vi "AlliGator Subtract Background Image(s) v4.vi"(8 "error in (no error)":errorcluster, 9 "Background Gate Images, Min, Max & Sum 2":T1, 10 "Background Gate Images, Min, Max & Sum 1":T1, 11 "AlliGator IV DVR in":refnum<data-value>) -> (0 "error out":errorcluster, 3 "AlliGator IV DVR out":refnum<data-value>)   [LabVIEW 2021, in "AlliGator Files.lvlib"]
doc: "Computes background-subtracted single- or dual-channel dataset image structures."
uses:
  AlliGator Files.lvlib
  Internal Variables/AlliGator Internal Variables v2.ctl
  <vilib>/vision/Image Controls.llb/IMAQ Image.ctl
  Internal Variables/AlliGator Gate Image Set.ctl
  AlliGator FLI Dataset Type.ctl
  AlliGator Data Series Type.ctl
  Dual-Channel Datasets/AlliGator Dataset Channel.ctl
  Settings/AlliGator Gate Arithmetic.ctl
  Source Image/AlliGator Displayed Image.ctl
  Image/Named ROI Description.ctl
  Phasor Graph/AlliGator Decay Metadata v3.ctl
  Decay Analysis/Decay Preprocessing/AlliGator Decay Background Subtraction Info.ctl
  Decay Analysis/Decay Preprocessing/AlliGator Baseline Subtraction Method.ctl
  Graphs/XY Graph/XY Graph Plot Shift Parameters.ctl
  Graphs/XY Graph/XY Graph Plot Shift Method.ctl
  Decay Analysis/Decay Preprocessing/AlliGator Decay Extrapolation Parameters.ctl
  Phasor/Calibration Phasor (m, phi).ctl
  Phasor/Phasor Reference Series.ctl
  Phasor/Phasor Calibration Map v2.ctl
  Phasor/Phasor (g, s).ctl
  Phasor Graph/AlliGator Raw Phasor Plot Data v5.ctl
  Phasor/Phasor Standard Deviation Options.ctl
  Phasor Plot/AlliGator Phasor Multi-Harmonic Data.ctl
  Phasor/Phasor Harmonic Data.ctl
  Decay Fit Parameter Map/AlliGator Decay Fit Options & Parameters v4.ctl
  Fits/IRF(X)PSED/Decay Fit Options v4.ctl
  Fits/Decay Convolution/Decay Model.ctl
  Fits/Residual Type.ctl
  Fits/IRF(X)PSED/Fit Weights Type v2.ctl
  Fits/Non-linear Fitting Method v2.ctl
  Fits/Fit Calculation Method.ctl
  Fits/Non-linear Fitting Algorithm.ctl
  Decay Analysis/Decay Fit/AlliGator Decay Fit Parameter Constraints 2.ctl
  Fits/IRF(X)PSED/Decay Fit Parameters In List.ctl
  Fits/IRF(X)PSED/MLE Baseline Offset Type.ctl
  Decay Analysis/Decay Preprocessing/AlliGator Decay Preprocessing Parameters.ctl
  Fits/IRF(X)PSED/Decay Fit Parameters & Derived Quantities List v2.ctl
  Fits/IRF(X)PSED/Decay Fit Result Constraint.ctl
  Decay Fit Parameter Map/AlliGator Parameter Maps Data.ctl
  Globals, Variables, Constants/AlliGator Variables List.ctl
  Variant/Variant to Data/Variant to U16.vi
  <vilib>/Utility/error.llb/Error Cluster From Error Code.vi
  <vilib>/ErrorRing/Error Ring.xnode
  <vilib>/vision/NI_Vision_Development_Module.lvlib
  Image/Image.lvlib
  Error/Error.lvlib
  Strings/Strings.lvlib
  Globals, Variables, Constants/AlliGator Globals, Variables & Constants.lvlib
  Dual-Channel Datasets/AlliGator Dual-Channel Datasets.lvlib
  Variant/Variant to Data/Variant to Data.lvlib
  Phasor/Phasor.lvlib
  Internal Variables/AlliGator Internal Variables.lvlib
  Phasor Graph/AlliGator Phasor Graph.lvlib
  Decay Analysis/Decay Preprocessing/AlliGator Decay Preprocessing.lvlib
  Graphs/XY Graph/XY Graph Add-Ons.lvlib
  Phasor Plot/AlliGator Phasor Plot.lvlib
  Source Image/AlliGator Source Image.lvlib
  Fits/Fits.lvlib
  Decay Analysis/Decay Fit/AlliGator Decay Fit.lvlib
  Settings/AlliGator Settings.lvlib
  Decay Fit Parameter Map/AlliGator Decay Fit Parameter Map.lvlib
panel:
  # "see the AlliGator License on the block diagram (Ctrl+E or Window:Show Block Diagram)"
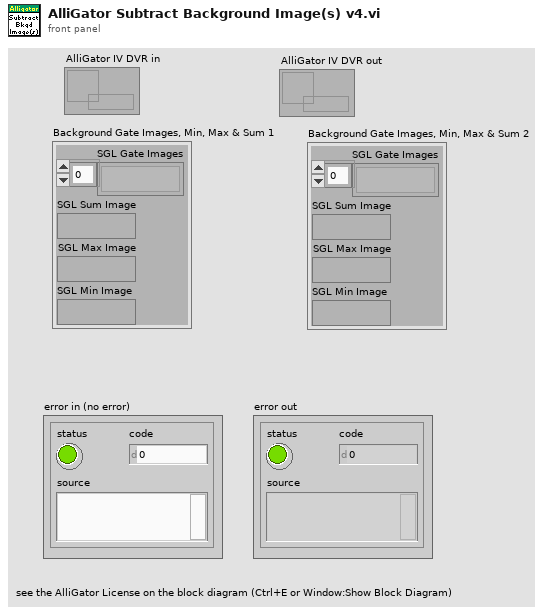
[diagram p1: front panel]
types:
  T1 = typedef "AlliGator Internal Variables.lvlib/AlliGator Gate Image Set.ctl" = cluster{"SGL Gate Images":T2[], "SGL Sum Image":T2, "SGL Max Image":T2, "SGL Min Image":T2}
  T2 = typedef "IMAQ Image.ctl" = refnum<image>
  T3 = typedef "Image Type" = u32
  T4 = typedef "AlliGator Globals, Variables & Constants.lvlib/AlliGator Variables List.ctl" = enum16{"---- GUI ----", "GUI:Initialization Status", "GUI:State Indicators Refnum", "GUI:Original AlliGator Menu Items", "GUI:Current Action Loop State", "GUI:Script in progress", "GUI:Playback", "GUI:Loop Playback", "GUI:Search ROI Used", "GUI:Search ROI", "Decay Graph Max Legend Size", "Intensity Graph Max Legend Size", "Decay Statistics Graph Max Legend Size", "Phasor Graph Max Legend Size", "Phasor Ratio Graph Max Legend Size", "Lifetime Graph Max Legend Size", "---- Files ----", "Files:Export Dataset Frames as Individual Files", "Files:Show Batch Export Help Balloons", "Files:Frames in Dataset", "Files:ptu File Frame Start Indices", "Files:Current Frame in Dataset", "Files:Current Frame Timestamp", "Files:Dataset Loaded", "Files:Dataset Metadata", "Files:Dataset Channel", "Files:Dataset Data Description", "Files:Background Dataset Metadata", "Files:Background Dataset Channel", "Files:Background Dataset Data Description", "Files:Background File Subtraction", "Files:Background File Path", "Files:Background File Pile-up Correction", "Files:Background File Pixel Well Capacity", "Files:Background File Scaling Factor", "Files:Current Dataset Load Settings", "Files:Dataset Path", "Files:ICCD-specific Information", "Files:Macrotime Gate Separation", "------ Python Plugins ------", "Python Plugins:Information", "Python Plugins:Python Session", "Python Plugins:Valid Python Session?", "---- Source Image ----", "Source Image:ROIs", "Source Image:Current ROI", "Source Image:ROI Event Refnum", "X_Source Image:Display Range", "X_Source Image:Palette Information", "X_Source Image:Type of Displayed Image", "X_Time Gate Slider", "Source Image:Palette List", "Source Image:Scale", "Source Image:ROI Overlay Color", "Source Image:Overlay to Erase", "Source Image:Is Displayed Image Accumulated", "Source Image:White Light Image Modified", "Source Image:Mask Image Modified", "---- Image Profile Window ----", "Image Profile:Window Event Refnum", "Image Profile:IntensityType", "Image Profile:Intensity Average Type", "Image Profile:Intensity-weighted SDV", "Image Profile:Box Profile Type", "Image Profile:Window Open", "Image Profile:Plotted Fit Parameter", "------ Phasor Graph -------", "Phasor Graph:Show Line", "---- Phasor Plot ---", "Phasor Plot:Parameters Changed", "Phasor Plot:FLI Dataset Modified since last Calculation", "Phasor Harmonics Data", "Selected Phasor Harmonics", "Phasor Harmonic Manager Event Refnum", "Phasor Plot:ROIs", "Phasor Plot:Current ROI", "Phasor Plot:ROI Event Refnum", "Phasor Plot:Image Reference Points", "Phasor Plot:Computed", "Phasor Plot:Palette Information", "Phasor Plot:Palette List", "Phasor Plot:Phasor Ratio Palette Information", "Phasor Plot:Phasor Ratio Palette List", "Phasor Plot:Image Scale", "Phasor Plot:Image Overlay to Erase", "Phasor Plot:Image Elements to Update", "Phasor Plot:Current Calculation Parameters", "Phasor Plot:Current Calibration Options", "Phasor Plot:Reset Cumulated Phasor Plot", "Phasor Plot:Reference 1", "Phasor Plot:Lifetime Reference 1", "Phasor Plot:Reference 1 Frequency", "Phasor Plot:Reference 2", "Phasor Plot:Lifetime Reference 2", "Phasor Plot:Reference 2 Frequency", "---- Decay Analysis ----", "Number of Selected Decays to Fit", "LS Fit Results", "LAR Fit Results", "BS Fit Results", "Last Decay Max - Min", "Best Fit Parameters", "Best Fit Parameter Names", "Actual Size X", "Actual Size Y", "Binning X", "Binning Y", "Actual # Gates", "Dataset Number", "Gates to...", "Gates Skipped", "Gates to keep", "Gate Step", "Gate Separation", "Reversed Gates", "Pile-up Correction", "Pixel Well Capacity", "Background Subtracted", "Background Subtraction Method", "Background Definition Range", "Background File (deprecated)", "Number of Dataset Accumulated", "Array of Accumulated Dataset Paths", "Do Averaged Datasets", "Destination File Path", "Process Plot Target", "Use 1/D as Phasor Frequency", "---- Decay Fit Parameter Map -----", "Decay Fit Parameter Map:Palette Information", "Decay Fit Parameter Map:Palette List", "Decay Fit Parameter Map:X Resolution", "Decay Fit Parameter Map:Y Resolution", "Decay Fit Parameter Map:Use Decay Fit Result Constraints", "Decay Fit Parameter Map:Decay Fit Result Constraints", "Decay Fit Parameter Map:Decay Fit Result Constraints Applied", "---- Parameter Map ----", "Parameter Map:Palette Information", "Parameter Map:Palette List", "------- Local Decay Window ---------", "Local Decay Graph Window:Event Refnum", "Local Decay Graph Window:Use normalized IRF for convolution", "----- Miscellaneous ----", "Misc:Skippable Dialog Windows Status"}
  T5 = typedef "AlliGator Internal Variables.lvlib/AlliGator Internal Variables v2.ctl" = cluster{"----------------------------- Images -----------------------------":u8, "Displayed Image":T2, "White Light Image":T2, "Mask Image":T2, "ROI Mask Image":T2, "Current Dataset Images 1":T1, "Background Dataset Images 1":T1, "Current Dataset Images 2":T1, "Background Dataset Images 2":T1, "Current Dataset Arithmetic Images":T1, "Accumulated Dataset Images 1":T1, "Accumulated Dataset Images 2":T1, "Accumulated Dataset Arithmetic Images":T1, "----------------------------- File Paths -----------------------------":u8, "Phasor Plot Image":T2, "Decay Fit Parameter Map Image":T2, "Parameter Map Image":T2, "Single Data Point Path":path, "White Light Image Path":path, "Mask Image Path":path, "Time-Series Folder":path, "[Time-Series Paths]":path[], "----------------------------- FLI Dataset -----------------------------":u8, "Current Dataset":i32, "Single Dataset Type":T6, "Current Folder":string, "AlliGator Data Series Type":T7, "# Datasets":i32, "Dual-Channel Dataset":bool, "Selected Channel Name":string, "Dataset Channel":T8, "Channel Arithmetic":T9, "Dual-Channel Background Dataset":bool, "Background Channel":T8, "Dual-Channel Accumulated Dataset":bool, "Start Time":dbl, "[Time-Series Timestamps]":dbl[], "[Intensity Corrections]":dbl[], "Time Series Script":bool, "Type of Displayed Image":T10, "Gate Image Slide":u16, "# Gates":i32, "ROIs":T11[], "----------------------------- Decays -----------------------------":u8, "ROI Decay":cluster{"t Array":dbl[], "I Array":dbl[]}, "Valid Decay":bool, "Decay  Metadata":T13, "Reference Decay Plot Name":string, "Reference Decay":cluster{"t Array":dbl[], "I Array":dbl[]}, "Decay Shift Plot":cluster{"Time Stamps":dbl[], "Decay Shifts":dbl[]}, "[Decays Max Values]":sgl[], "[Decays Min Values]":sgl[], "----------------------------- Calibration -----------------------------":u8, "Calibration Phasor":T19, "Calibration Phasor Series":T20, "Phasor Calibration Map":T21, "Calibration Map MD5 Digest":string, "----------------------------- Phasor Graph -----------------------------":u8, "Last Raw Phasor":T22, "Last Calibrated Phasor":T22, "Last Calibrated Phasor SDV":T22, "Phasor Graph:Phasor Plot":cluster{"g Array":dbl[], "s Array":dbl[]}, "Phasor Graph:Phasor SDV Plot":cluster{"g Array":dbl[], "s Array":dbl[]}, "[Phasor Graph:Raw Phasor Plots]":T23[], "Phasor Plot locked to Ref 1":i32, "[Phasor Plot(s) locked to Ref 1]":i32[], "[Phasor Plot(s) locked to Ref 2]":i32[], "[Pixel Phasors]":T22[], "----------------------------- Phasor Plot -----------------------------":u8, "[[Sum Image]]":dbl[][], "[[CSG Phasors]]":csg[][], "[[Valid Pixel?]]":bool[][], "[[Phasor Ratios]]":dbl[][], "[[Average Lifetimes]]":dbl[][], "Amplitude Weighted Average Lifetime":bool, "I/m/phi Dataset":cluster{"I/m/phi Dataset?":bool, "Base Frequency":dbl[unit], "Harmonic Orders":u8[]}, "Multi Phasor Plot Data":T25, "----------------------------- Decay Fit Parameter Map -----------------------------":u8, "Decay Fit Options & Parameters":T27, "Fit Options: Decay Preprocessing Parameters":T38, "Fit Options: Reference Decay":cluster{"t Array":dbl[], "I Array":dbl[]}, "Is Full Image Parameters Map":bool, "Is Single-Pixels Parameters Map":bool, "NLSF Parameters Map X Resolution":i32, "NLSF Parameters Map Y Resolution":i32, "[Single Decay Fit Parameters]":dbl[], "Fit Model":T29, "[[Multiple Decays Fit Parameters]]":dbl[][], "[[Multiple Decays Fit Parameter SDVs]]":dbl[][], "[[IRFs]]":dbl[][], "[ROI Descriptors]":T12[], "IRF Array Time Axis":dbl[], "Decay Array Time Axis":dbl[], "[Decay Fit Parameter Names]":T39[], "[Decay Sum]":dbl[], "Array of Decay Fit Result Constraints":T40[], "Selected ROIs Array":bool[], "----------------------------- Parameter Maps -----------------------------":u8, "[Map Set Names]":string[], "[Parameter Maps]":T41[], "[[User-defined Quantities]]":dbl[][], "User-defined Quantity":string}
  T6 = typedef "AlliGator Files.lvlib/AlliGator FLI Dataset Type.ctl" = enum16{"HDF5 FLI Dataset", "Gate Image Folder", ".sdt FLI Dataset (Becker & Hickl)", ".ptu FLI Dataset (PicoQuant)", "SS1 FLI Dataset", "SS2 FLI Dataset", "I/m/phi Dataset", ".bin FLI Dataset (PicoQuant Binned)", ".bin FLI Dataset (Piccolo Binned)", ".mat FLI Dataset"}
  T7 = typedef "AlliGator Files.lvlib/AlliGator Data Series Type.ctl" = enum16{"Not a Supported Series", "Gate Images Folder Series", "SwissSPAD 2 Dataset Series", "B&H FLI Dataset Series", "PicoQuant PTU FLI Dataset Series", "PicoQuant BIN FLI Dataset Series", "Piccolo hist BIN FLI Dataset Series", "HDF5 FLI Dataset Series"}
  T8 = typedef "AlliGator Dual-Channel Datasets.lvlib/AlliGator Dataset Channel.ctl" = enum16{"G2", "INT"}
  T9 = typedef "AlliGator Settings.lvlib/AlliGator Gate Arithmetic.ctl" = enum16{"None", "INT-G2", "G2/INT*<INT>", "(1 - G2/INT)*<INT>"}
  T10 = typedef "AlliGator Source Image.lvlib/AlliGator Displayed Image.ctl" = enum16{"Single Gate", "Sum of All Gates", "Max of All Gates", "Min of All Gates", "-", "White Ligth Image", "Mask Image"}
  T11 = typedef "Image.lvlib/Named ROI Description.ctl" = cluster{"ROI Descriptor":T12, "ROI Name":string, "Overlay Color":u32}
  T12 = typedef "ROI Descriptor" = cluster{"Global Rectangle":i32[], "Contours":cluster{"ID":enum32{"External", "Internal"}, "Type":u32, "Coordinates":i32[]}[]}
  T13 = typedef "AlliGator Phasor Graph.lvlib/AlliGator Decay Metadata v3.ctl" = cluster{"ROI Descriptor":T12, "ROI Center":cluster{"X":i32, "Y":i32}, "Decay Background Subtraction Info":T14, "Decay Reverted":bool, "Decay Smoothened":bool, "Decay Straightened":bool, "Fitted Tau (Decay Straightening)":dbl, "Decay Shift Parameters":T16, "Decay Shifted":bool, "Decay Extrapolated":bool, "Decay Extrapolation Parameters":T18, "Decay Normalized":bool, "Fold Decay":bool, "# Folds":u32}
  T14 = typedef "AlliGator Decay Preprocessing.lvlib/AlliGator Decay Background Subtraction Info.ctl" = cluster{"Laser Period":dbl[unit], "Gate Duration":dbl[unit], "Baseline Subtraction Method":T15, "Background Definition Range":cluster{"Min Gate":dbl[unit], "Max Gate":dbl[unit]}, "Total Intensity w/o Bkgd Subtraction":dbl, "Bkgd-subtracted Intensity (exp)":dbl, "# Data Points":i32, "Background/Gate":dbl, "Fitted Lifetime":dbl[unit], "Bkgd-subtracted Intensity (theo)":dbl}
  T15 = typedef "AlliGator Decay Preprocessing.lvlib/AlliGator Baseline Subtraction Method.ctl" = enum16{"Mean", "Min", "Square Gated Single-Exponential", "File", "Constant"}
  T16 = typedef "XY Graph Add-Ons.lvlib/XY Graph Plot Shift Parameters.ctl" = cluster{"Type":T17, "Shift":dbl[unit], "Threshold":dbl, "Rotate":bool}
  T17 = typedef "XY Graph Add-Ons.lvlib/XY Graph Plot Shift Method.ctl" = enum16{"Default", "CFD", "Threshold", "Cross-Correlation"}
  T18 = typedef "AlliGator Decay Preprocessing.lvlib/AlliGator Decay Extrapolation Parameters.ctl" = cluster{"Additional Points":u32, "Head Fraction":dbl, "Fitted Tau":dbl, "Use Periodicity":bool, "Use Cursors":bool, "Tail Fraction":dbl}
  T19 = typedef "Phasor.lvlib/Calibration Phasor (m, phi).ctl" = cluster{"m":dbl, "phi":dbl, "Phasor Frequency":dbl[unit], "Reference Lifetime":dbl[unit]}
  T20 = typedef "Phasor.lvlib/Phasor Reference Series.ctl" = cluster{"m Array":dbl[], "phi Array":dbl[], "Phasor Frequency":dbl[unit], "Calibration Lifetime":dbl[unit]}
  T21 = typedef "Phasor.lvlib/Phasor Calibration Map v2.ctl" = cluster{"Phasor Frequency":dbl[unit], "Calibration Lifetime":dbl[unit], "ROI Centers":cluster{"X":i32, "Y":i32}[], "ROI Descriptors":T12[], "Map Resolution X":i32, "Map Resolution Y":i32, "z Array":cdb[]}
  T22 = typedef "Phasor.lvlib/Phasor (g, s).ctl" = cluster{"g":dbl, "s":dbl}
  T23 = typedef "AlliGator Phasor Graph.lvlib/AlliGator Raw Phasor Plot Data v5.ctl" = cluster{"Phasor Plot Name":string, "Raw Phasor Plot":T22[], "Phasor Frequency":dbl[unit], "[Decay Metadata]":T13[], "Raw Phasor Plot SDV":T22[], "Phasor SDV Options":T24, "[Calibration Phasor]":T19[], "Intensity Array":dbl[]}
  T24 = typedef "Phasor.lvlib/Phasor Standard Deviation Options.ctl" = cluster{"Compute Estimated SDV":bool, "# Replicas":u32, "Use Estimated Average Phasor":bool}
  T25 = typedef "AlliGator Phasor Plot.lvlib/AlliGator Phasor Multi-Harmonic Data.ctl" = cluster{"Base Frequency":dbl[unit], "# Harmonics":u8, "Harmonic Orders":u8[], "Phasor Plot Settings Checksum":u64, "Phasor Harmonic Data Array":T26[]}
  T26 = typedef "Phasor.lvlib/Phasor Harmonic Data.ctl" = cluster{"Phasor Harmonic Name":string, "Phasor Plot Settings Checksum":u64, "Phasor Frequency":dbl[unit], "Base Frequency":dbl[unit], "Harmonic Order":u8, "Phasor Plot Parameters":string, "Phasor Array [[CSG]]":csg[][], "Dataset File Path":path}
  T27 = typedef "AlliGator Decay Fit Parameter Map.lvlib/AlliGator Decay Fit Options & Parameters v4.ctl" = cluster{"SYNC Period":dbl[unit], "Fit Options":T28, "Fit Parameter Constraints":T35[], "MLE Baseline Offset":dbl, "MLE Baseline Offset Type":T37}
  T28 = typedef "Fits.lvlib/Decay Fit Options v4.ctl" = cluster{"Show Fit Residuals":bool, "Fit Model":T29, "Residual Type":T30, "Max Decay Percentile":dbl, "Min Decay Percentile":dbl, "Show Full Decay":bool, "Weights":T31, "Fitting Method":T32, "Compute Parameter Uncertainties":bool, "Periodic Boundaries":bool, "Model Calculation":T33, "Period":dbl[unit], "Termination Criteria":cluster{"Max Iterations":i32, "Max Function Calls":i32, "Max Time":dbl[unit], "Function Tolerance":dbl, "Parameter Tolerance":dbl, "Gradient Tolerance":dbl, "Min Lambda":dbl, "Max Lambda":dbl, "Initial Tick Count":u32}, "Offset Resolution":dbl[unit], "Use Local IRF":bool, "Fitting Algorithm":T34, "Show Confidence Interval ":bool, "Confidence Level":dbl}
  T29 = typedef "Fits.lvlib/Decay Model.ctl" = enum16{"1-Exponential", "2-Exponentials"}
  T30 = typedef "Fits.lvlib/Residual Type.ctl" = enum16{"Standard", "Normalized", "Reduced"}
  T31 = typedef "Fits.lvlib/Fit Weights Type v2.ctl" = enum16{"Unweighted", "1/Variance (Neyman)", "1/Variance (Pearson)", "Best of All"}
  T32 = typedef "Fits.lvlib/Non-linear Fitting Method v2.ctl" = enum16{"Least Square", "Least Absolute Residual", "Bisquare", "MLE", "-", "Best of All"}
  T33 = typedef "Fits.lvlib/Fit Calculation Method.ctl" = enum16{"Simulation", "Convolution", "Integration"}
  T34 = typedef "Fits.lvlib/Non-linear Fitting Algorithm.ctl" = enum16{"Levenberg-Marquardt", "Trust-Region Dogleg"}
  T35 = typedef "AlliGator Decay Fit.lvlib/AlliGator Decay Fit Parameter Constraints 2.ctl" = cluster{"Fit Parameter":T36, "Min Value":dbl, "Max Value":dbl, "Global":bool, "Used":bool}
  T36 = typedef "Fits.lvlib/Decay Fit Parameters In List.ctl" = enum16{"Offset", "Baseline", "A_1", "tau_1", "A_2", "tau_2"}
  T37 = typedef "Fits.lvlib/MLE Baseline Offset Type.ctl" = enum32{"Absolute", "Percentage"}
  T38 = typedef "AlliGator Decay Preprocessing.lvlib/AlliGator Decay Preprocessing Parameters.ctl" = cluster{"Background Subtraction":bool, "Straighten Decay":bool, "Reverse Gates":bool, "1-Normalized Decay":bool, "Smoothen Decay":bool, "Smoothing Parameter":dbl, "Shift Decay":bool, "Decay Shift Parameters":T16, "Extrapolate Decay":bool, "Additional Points":u32, "Head Fraction":dbl, "Pixel-Normalize Decay":bool, "Use Periodicity":bool, "Use Cursors":bool, "Tail Fraction":dbl, "Use Decay Pre-Processing":bool, "Fold Decay":bool, "# Folds":u32, "[0-1]-Normalized Decay":bool}
  T39 = typedef "Fits.lvlib/Decay Fit Parameters & Derived Quantities List v2.ctl" = enum16{"Offset", "Baseline", "A_1", "tau_1", "A_2", "tau_2", "<tau>_a", "f1_a", "f2_a", "<tau>_i", "f1_i", "f2_i", "-", "R^2", "Chi^2"}
  T40 = typedef "Fits.lvlib/Decay Fit Result Constraint.ctl" = cluster{"Fit Parameter":enum16{"Offset", "Baseline", "A_1", "tau_1", "A_2", "tau_2", "<tau>_a", "f1_a", "f2_a", "<tau>_i", "f1_i", "f2_i", "-", "R^2", "Chi^2", "Max Relative Residual", "<Residual ACF>", "Residual ACF SDV", "tau_2/tau_1"}, "Min Value":dbl, "Max Value":dbl, "Use Constraint":bool}
  T41 = typedef "AlliGator Decay Fit Parameter Map.lvlib/AlliGator Parameter Maps Data.ctl" = cluster{"Map Set Name":string, "[Parameter Names]":string[], "[[Parameters]]":dbl[][], "[[Parameter SDVs]]":dbl[][], "Decay Array Time Axis":dbl[], "[[IRFs]]":dbl[][], "IRF Array Time Axis":dbl[], "X Resolution":i32, "Y Resolution":i32, "Intensity Array":dbl[]}
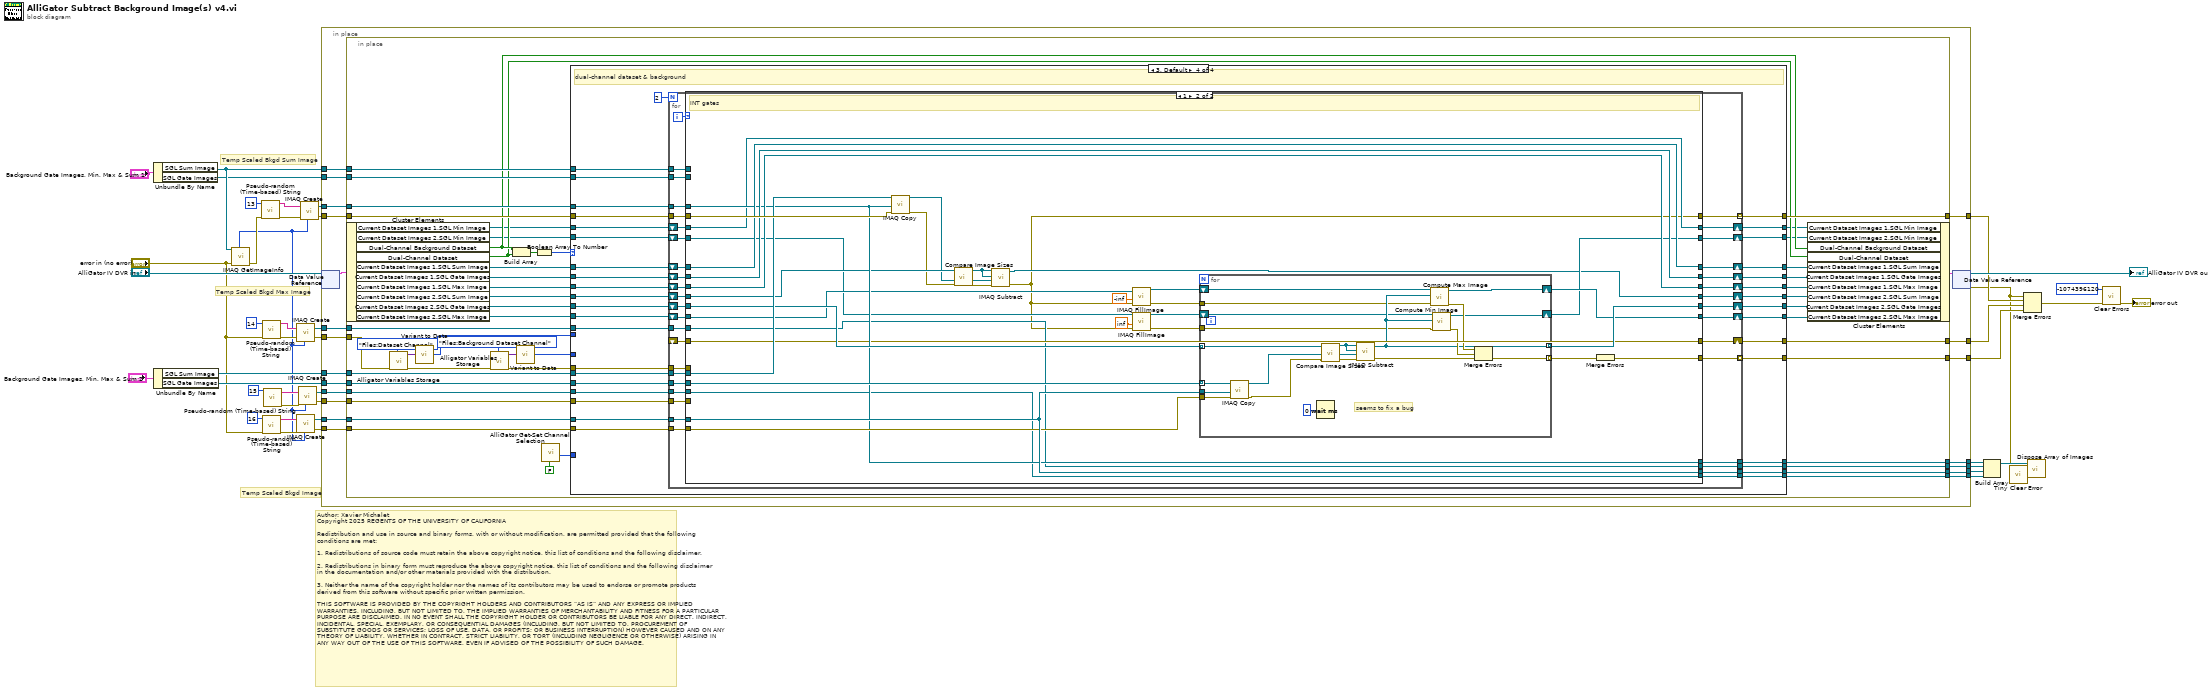
[diagram p0: block diagram]
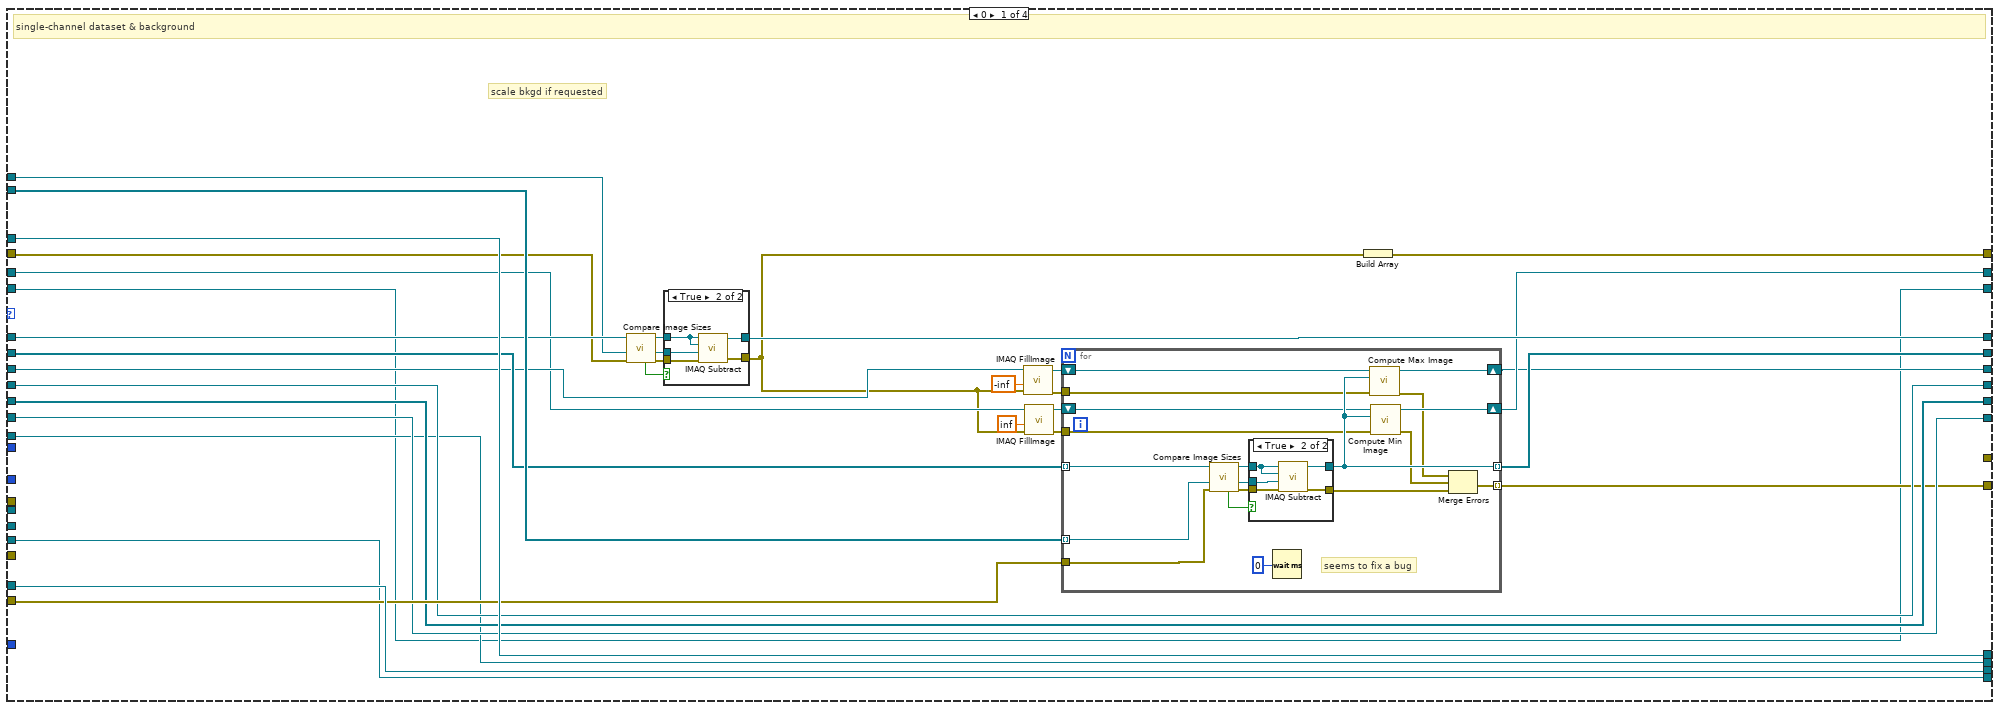
[diagram p2: hidden frame]
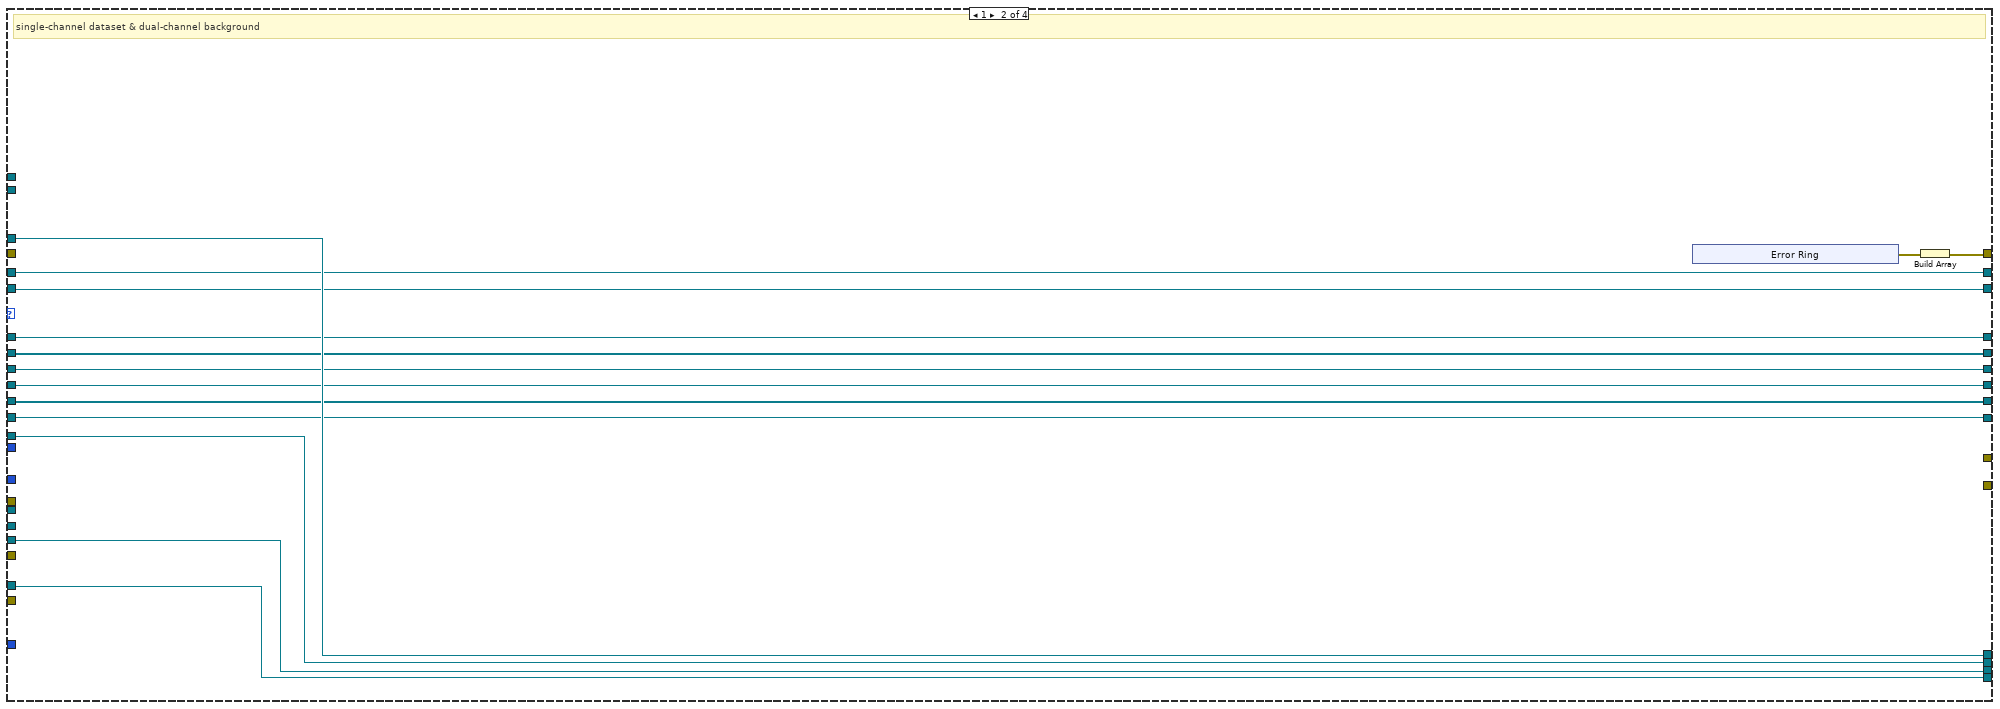
[diagram p5: hidden frame]
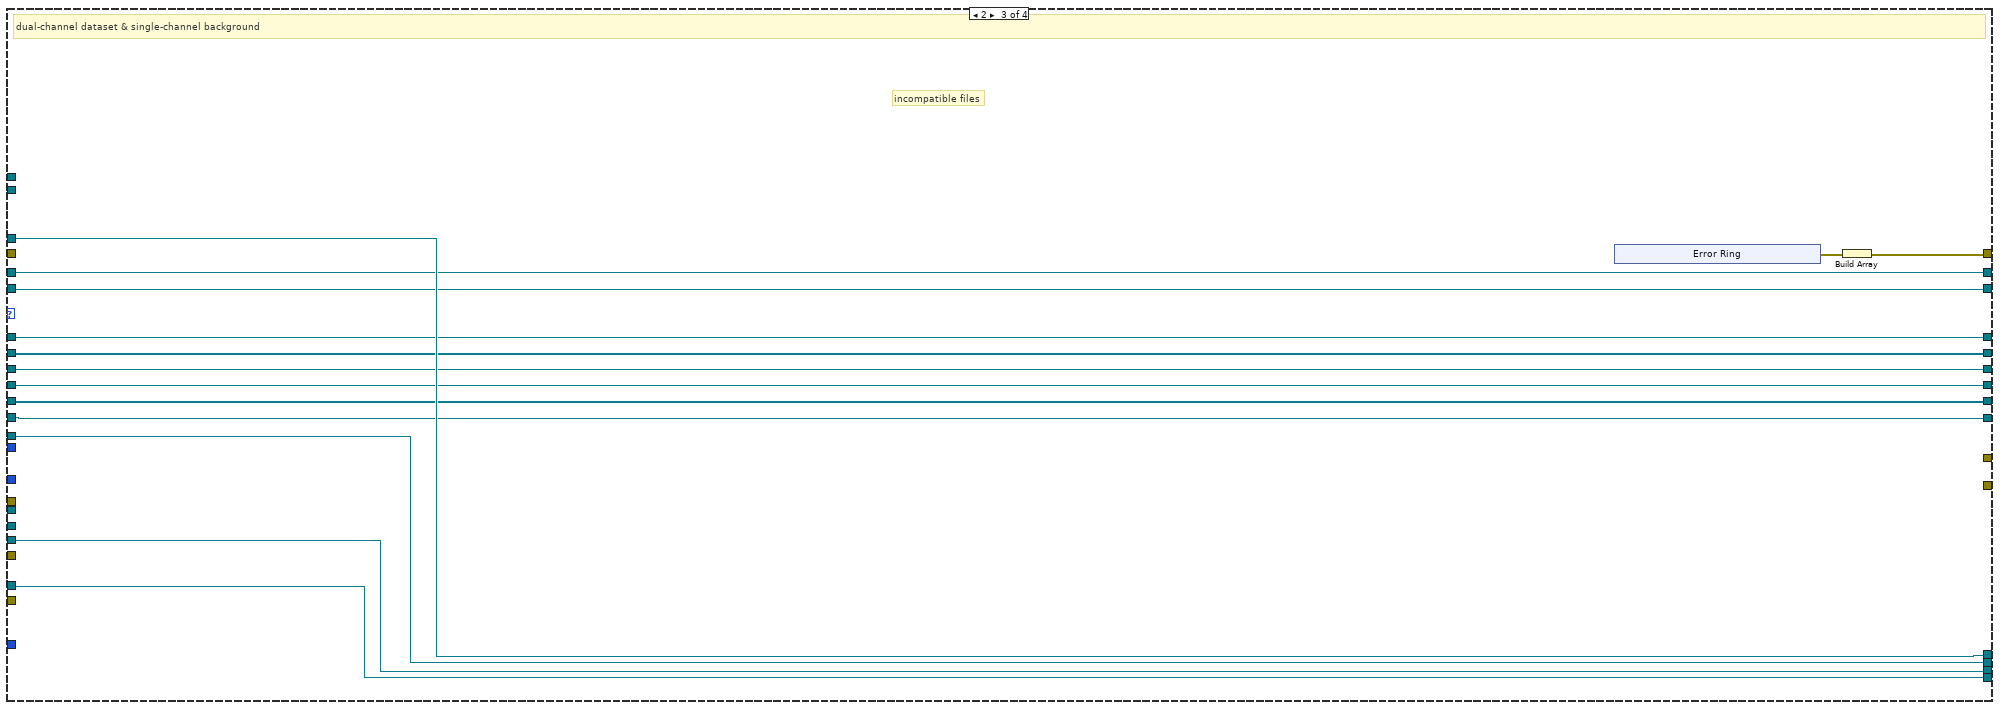
[diagram p6: hidden frame]
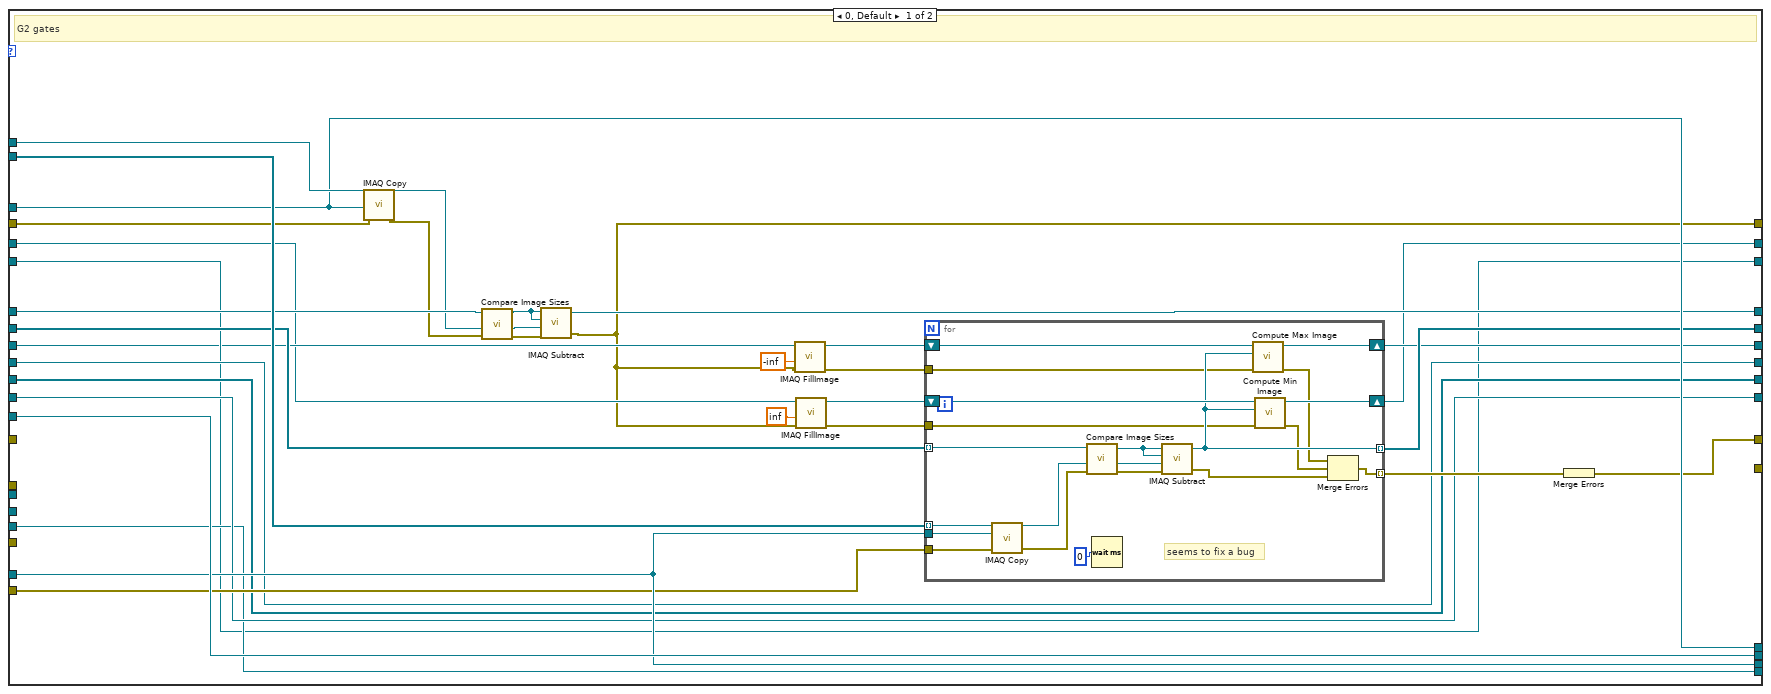
[diagram p7: hidden frame]
diagram:
  # "Author: Xavier Michalet\nCopyright 2025 REGENTS OF THE UNIVERSITY OF CALIFORNIA\n\nRedistribution and use in source and binary forms, with or without modification, are permitted provided that the following conditions are met:\n\n1. Redistributions of source code must retain the above copyright notice, this list of conditions and the following disclaimer.\n\n2. Redistributions in binary form must reproduce the above copyright notice, this list of conditions and the following disclaimer in the documentation and/or other materials provided with the distribution.\n\n3. Neither the name of the copyright holder nor the names of its contributors may be used to endorse or promote products derived from this software without specific prior written permission.\n\nTHIS SOFTWARE IS PROVIDED BY THE COPYRIGHT HOLDERS AND CONTRIBUTORS “AS IS” AND ANY EXPRESS OR IMPLIED WARRANTIES, INCLUDING, BUT NOT LIMITED TO, THE IMPLIED WARRANTIES OF MERCHANTABILITY AND FITNESS FOR A PARTICULAR PURPOSE ARE DISCLAIMED. IN NO EVENT SHALL THE COPYRIGHT HOLDER OR CONTRIBUTORS BE LIABLE FOR ANY DIRECT, INDIRECT, INCIDENTAL, SPECIAL, EXEMPLARY, OR CONSEQUENTIAL DAMAGES (INCLUDING, BUT NOT LIMITED TO, PROCUREMENT OF SUBSTITUTE GOODS OR SERVICES; LOSS OF USE, DATA, OR PROFITS; OR BUSINESS INTERRUPTION) HOWEVER CAUSED AND ON ANY THEORY OF LIABILITY, WHETHER IN CONTRACT, STRICT LIABILITY, OR TORT (INCLUDING NEGLIGENCE OR OTHERWISE) ARISING IN ANY WAY OUT OF THE USE OF THIS SOFTWARE, EVEN IF ADVISED OF THE POSSIBILITY OF SUCH DAMAGE."
  # "Temp Scaled Bkgd Max Image"
  # "Temp Scaled Bkgd Image"
  # "Temp Scaled Bkgd Sum Image"
  n1 = Unbundle By Name("Background Gate Images, Min, Max & Sum 1") -> ("SGL Sum Image"=w41:T2, "SGL Gate Images"=w40:T2[])
  n2 = Unbundle By Name("Background Gate Images, Min, Max & Sum 2") -> ("SGL Sum Image"=w38:T2, "SGL Gate Images"=w37:T2[])
  n3 = call "IMAQ GetImageInfo"("error in (no error)"="error in (no error)", "Image"=w41) -> ("error out"=w15:errorcluster, "Image Type"=w5:T3)  [unwired: 2 in, 6 out]
  n4 = call "Pseudo-random (Time-based) String.vi"("Error In"=w15, "Length (10)"=u32 13) -> ("Error Out"=w20:errorcluster, "result string"=w22:string)  [unwired: 8 in]
  n5 = call "Pseudo-random (Time-based) String.vi"("Error In"="error in (no error)", "Length (10)"=u32 14) -> ("Error Out"=w19:errorcluster, "result string"=w21:string)  [unwired: 8 in]
  n6 = call "Pseudo-random (Time-based) String.vi"("Error In"="error in (no error)", "Length (10)"=u32 16) -> ("Error Out"=w18:errorcluster, "result string"=w17:string)  [unwired: 8 in]
  n7 = call "Pseudo-random (Time-based) String.vi"("Length (10)"=u32 15) -> ("Error Out"=w6:errorcluster, "result string"=w7:string)  [unwired: 9 in]
  n8 = call "IMAQ Create"("Image Name"=w21, "Image Type"=w5, "error in (no error)"=w19) -> ("New Image"=w30:T2, "error out"=w25:errorcluster)  [unwired: 2 in]
  n9 = call "IMAQ Create"("Image Name"=w17, "Image Type"=w5, "error in (no error)"=w18) -> ("New Image"=w27:T2, "error out"=w24:errorcluster)  [unwired: 2 in]
  n10 = call "IMAQ Create"("Image Name"=w7, "Image Type"=w5, "error in (no error)"=w6) -> ("New Image"=w3:T2, "error out"=w4:errorcluster)  [unwired: 2 in]
  n11 = call "IMAQ Create"("Image Name"=w22, "Image Type"=w5, "error in (no error)"=w20) -> ("New Image"=w33:T2, "error out"=w32:errorcluster)  [unwired: 2 in]
  n12 = in-place {
    in-place-border: w41 -> [w65]
    in-place-border: w40 -> [w64]
    in-place-border: [w63] -> w36
    in-place-border: [w62] -> w35
    in-place-border: [w61] -> w34
    in-place-border: w33 -> [w58]
    in-place-border: w32 -> [w60]
    in-place-border: [w59] -> w31
    in-place-border: w30 -> [w57]
    in-place-border: [w56] -> w28
    in-place-border: w27 -> [w55]
    in-place-border: [w54] -> w26
    in-place-border: w25 -> [w53]
    in-place-border: w24 -> [w52]
    in-place-border: w38 -> [w51]
    in-place-border: w37 -> [w50]
    in-place-border: w4 -> [w47]
    in-place-border: w3 -> [w46]
    in-place-border: [w45] -> w2
    n13 = in-place-dvr #1("AlliGator IV DVR in") -> (w49:T5)  [unwired: 1 out]
    n14 = in-place {
      in-place-border: w65 -> [w114]
      in-place-border: w64 -> [w113]
      in-place-border: [w112] -> w63
      in-place-border: [w111] -> w62
      in-place-border: [w66] -> w61
      in-place-border: w60 -> [w110]
      in-place-border: [w109] -> w59
      in-place-border: w58 -> [w108]
      in-place-border: w57 -> [w107]
      in-place-border: [w106] -> w56
      in-place-border: w55 -> [w105]
      in-place-border: [w104] -> w54
      in-place-border: w53 -> [w76]
      in-place-border: w52 -> [w103]
      in-place-border: w51 -> [w102]
      in-place-border: w50 -> [w101]
      in-place-border: w47 -> [w70]
      in-place-border: w46 -> [w69]
      in-place-border: [w67] -> w45
      n15 = in-place-cluster #2(w49) -> ("Current Dataset Images 1.SGL Min Image"=w68:T2, "Current Dataset Images 2.SGL Min Image"=w73:T2, "Dual-Channel Background Dataset"=w88:bool, "Dual-Channel Dataset"=w87:bool, "Current Dataset Images 1.SGL Sum Image"=w100:T2, "Current Dataset Images 1.SGL Gate Images"=w99:T2[], "Current Dataset Images 1.SGL Max Image"=w98:T2, "Current Dataset Images 2.SGL Sum Image"=w94:T2, "Current Dataset Images 2.SGL Gate Images"=w93:T2[], "Current Dataset Images 2.SGL Max Image"=w89:T2)
      n16 = call "Alligator Variables Storage.vi"("AlliGator Variable"=AlliGator_Variables_List."Files:Dataset Channel" ("Alligator Variable"), "Error In"=w76) -> ("Error Out"=w78:errorcluster, "Data out"=w81:variant)  [unwired: 7 in, 1 out]
      n17 = call-poly "Variant to Data.vi"("Variant"=w81) -> ("U16 Value"=w75:u16)  [unwired: 8 in]
      n18 = call "Alligator Variables Storage.vi"("AlliGator Variable"=AlliGator_Variables_List."Files:Background Dataset Channel" ("Alligator Variable"), "Error In"=w78) -> ("Error Out"=w77:errorcluster, "Data out"=w79:variant)  [unwired: 7 in, 1 out]
      n19 = Build Array(w88, w87) -> (w86:bool[])
      n20 = call-poly "Variant to Data.vi"("Variant"=w79) -> ("U16 Value"=w74:u16)  [unwired: 8 in]
      n21 = Boolean Array To Number(Boolean array=w86) -> (number=w85:u32)
      n22 = call "AlliGator Get-Set Channel Selection.vi"("Set (T)/Get (F)"=FALSE) -> ("Channel Arithmetic"=w83:T9)  [unwired: 7 in, 3 out]
      n23 = case shown="3, Default" w85 {
        tunnel: w114 -> [w133 _ _ w251]
        tunnel: w113 -> [w146 _ _ w250]
        tunnel: [w130 _ _ w249] -> w112
        tunnel: [w129 w193 w211 w248] -> w111
        tunnel: w110 -> [w135 _ _ w247]
        tunnel: [w145 w192 w210 w246] -> w109
        tunnel: w108 -> [w145 w192 w210 w245]
        tunnel: w107 -> [w122 w191 w209 w244]
        tunnel: [w122 w191 w209 w243] -> w106
        tunnel: w105 -> [w144 w187 w207 w242]
        tunnel: [w144 w188 w208 w241] -> w104
        tunnel: w77 -> [_ _ _ w240]
        tunnel: w103 -> [w143 _ _ w239]
        tunnel: w102 -> [_ _ _ w238]
        tunnel: w101 -> [_ _ _ w237]
        tunnel: w100 -> [w142 w185 w203 w236]
        tunnel: w99 -> [w141 w184 w202 w235]
        tunnel: w98 -> [w118 w183 w201 w234]
        tunnel: [w140 w185 w203 w233] -> w97
        tunnel: [w139 w184 w202 w232] -> w96
        tunnel: [w127 w183 w201 w231] -> w95
        tunnel: w94 -> [w138 w182 w200 w230]
        tunnel: w93 -> [w137 w181 w199 w229]
        tunnel: [w138 w182 w200 w228] -> w92
        tunnel: [w137 w181 w199 w227] -> w91
        tunnel: [w136 w180 w198 w226] -> w90
        tunnel: w89 -> [w136 w180 w198 w224]
        tunnel: w83 -> [_ _ _ _]
        tunnel: w74 -> [_ _ _ _]
        tunnel: w75 -> [_ _ _ _]
        tunnel: w73 -> [w116 w189 w205 w218]
        tunnel: [w116 w189 w205 w216] -> w72
        tunnel: [w128 w190 w206 w220] -> w71
        tunnel: w70 -> [_ _ _ w223]
        tunnel: w69 -> [w119 w188 w208 w222]
        tunnel: w68 -> [w117 w190 w206 w219]
        tunnel: [w119 w187 w207 w221] -> w67
        tunnel: [_ _ _ w217] -> w66
        frame 0 {
          # "scale bkgd if requested"
          # "single-channel dataset & background"
          n24 = call "Compare Image Sizes.vi"("Image Refnum 2"=w133, "Image Refnum 1"=w142) -> ("Image Refnum 2 (dup)"=w132:T2, "Image Refnum 1 (dup)"=w134:T2, "Comparable Images?"=w131:bool)  [unwired: 6 in, 1 out]
          n25 = case shown="True" w131 {
            tunnel: [w148 w153] -> w140
            tunnel: w135 -> [w147 w152]
            tunnel: [w147 w151] -> w115
            tunnel: w134 -> [w148 w150]
            tunnel: w132 -> [_ w149]
            frame False {
            }
            frame True {
              n26 = call "IMAQ Subtract"("Image Src A"=w150, "Image Dst"=w150, "Image Src B"=w149, "error in (no error)"=w152) -> ("Image Dst Out"=w153:T2, "error out"=w151:errorcluster)  [unwired: 3 in]
            }
          }
          n27 = call "IMAQ FillImage"("error in (no error)"=w115, "Pixel Value (U8, U16, I16, Float)"=sgl -inf, "Image"=w118) -> ("error out"=w121:errorcluster, "Image Out"=w124:T2)  [unwired: 7 in]
          n28 = call "IMAQ FillImage"("error in (no error)"=w115, "Pixel Value (U8, U16, I16, Float)"=sgl inf, "Image"=w117) -> ("error out"=w120:errorcluster, "Image Out"=w126:T2)  [unwired: 7 in]
          n29 = for {
            tunnel: w141 -> [w170] mode=indexing
            tunnel: w146 -> [w171] mode=indexing
            tunnel: [w162] -> w139 mode=indexing
            tunnel: [w159] -> w130 mode=indexing
            tunnel: w143 -> [w172]
            shift-right: [w163] -> w127
            shift-left: w124 -> [w164]
            shift-right: [w161] -> w128
            shift-left: w126 -> [w157]
            tunnel: w121 -> [w156]
            tunnel: w120 -> [w155]
            # "seems to fix a bug"
            n30 = call "Compare Image Sizes.vi"("error in (no error)"=w172, "Image Refnum 2"=w171, "Image Refnum 1"=w170) -> ("error out"=w167:errorcluster, "Image Refnum 2 (dup)"=w168:T2, "Image Refnum 1 (dup)"=w169:T2, "Comparable Images?"=w166:bool)  [unwired: 5 in]
            n31 = case shown="True" w166 {
              tunnel: [w174 w179] -> w162
              tunnel: [w173 w178] -> w154
              tunnel: w169 -> [w174 w177]
              tunnel: w168 -> [_ w176]
              tunnel: w167 -> [w173 w175]
              frame False {
              }
              frame True {
                n32 = call "IMAQ Subtract"("Image Src A"=w177, "Image Dst"=w177, "Image Src B"=w176, "error in (no error)"=w175) -> ("Image Dst Out"=w179:T2, "error out"=w178:errorcluster)  [unwired: 3 in]
              }
            }
            n33 = Wait (ms)(milliseconds to wait=u32 0) -> ()  [unwired: 1 out]
            n34 = call "Compute Max Image.vi"("error in (no error)"=w156, "New Image"=w162, "Max Image Dst"=w164) -> ("error out"=w160:errorcluster, "Max Image"=w163:T2)  [unwired: 7 in]
            n35 = call "Compute Min Image.vi"("error in (no error)"=w155, "New Image"=w162, "Min Image Dst"=w157) -> ("error out"=w158:errorcluster, "Min Image"=w161:T2)  [unwired: 7 in]
            n36 = Merge Errors(w160, w158, w154) -> (w159:errorcluster)
          }
          n37 = Build Array(w115) -> (w129:errorcluster[])
        }
        frame 1 {
          # "single-channel dataset & dual-channel background"
          n38 = xnode "Error Ring"() -> ("error out"=w186:errorcluster)
          n39 = Build Array(w186) -> (w193:errorcluster[])
        }
        frame 2 {
          # "incompatible files"
          # "dual-channel dataset & single-channel background"
          n40 = xnode "Error Ring"() -> ("error out"=w204:errorcluster)
          n41 = Build Array(w204) -> (w211:errorcluster[])
        }
        frame 3, Default {
          # "dual-channel dataset & background"
          n42 = for {
            N: 2 -> [_]
            tunnel: w250 -> [w287]
            tunnel: w244 -> [w281]
            tunnel: w242 -> [w279]
            tunnel: w238 -> [w274]
            tunnel: w251 -> [w288]
            tunnel: [w283] -> w246
            tunnel: w245 -> [w282]
            tunnel: [w278] -> w241
            tunnel: [w280] -> w243
            tunnel: w237 -> [w273]
            shift-right: [w265] -> w233
            shift-left: w236 -> [w272]
            shift-right: [w264] -> w232
            shift-left: w235 -> [w261]
            shift-right: [w263] -> w231
            shift-left: w234 -> [w271]
            shift-right: [w268] -> w228
            shift-left: w230 -> [w270]
            shift-right: [w267] -> w227
            shift-left: w229 -> [w269]
            shift-right: [w266] -> w226
            shift-left: w224 -> [w262]
            tunnel: w247 -> [w284]
            tunnel: [w285] -> w248 mode=indexing
            tunnel: w240 -> [w277]
            tunnel: [w286] -> w249 mode=indexing
            tunnel: w239 -> [w276]
            tunnel: w223 -> [w260]
            tunnel: w222 -> [w259]
            tunnel: [w258] -> w221
            shift-right: [w257] -> w220
            shift-left: w219 -> [w255]
            shift-right: [w256] -> w216
            shift-left: w218 -> [w252]
            shift-right: [w254] -> w217
            shift-left: _ -> [w253]
            i -> [w275]
            n43 = case shown="1" w275 {
              tunnel: w288 -> [w322 _]
              tunnel: w287 -> [w321 _]
              tunnel: w262 -> [w310 w346]
              tunnel: [_ w366] -> w286
              tunnel: [w289 w344] -> w285
              tunnel: w284 -> [w320 w378]
              tunnel: [w319 w367] -> w283
              tunnel: w282 -> [w319 w367]
              tunnel: w281 -> [w318 w347]
              tunnel: [w318 w347] -> w280
              tunnel: w279 -> [w317 w377]
              tunnel: [w317 w377] -> w278
              tunnel: w277 -> [_ _]
              tunnel: w276 -> [w316 w376]
              tunnel: w274 -> [_ w375]
              tunnel: w273 -> [_ w374]
              tunnel: w272 -> [w309 w370]
              tunnel: w271 -> [w291 w368]
              tunnel: w270 -> [w312 w365]
              tunnel: w269 -> [w311 w373]
              tunnel: [w312 w352] -> w268
              tunnel: [w311 w371] -> w267
              tunnel: [w310 w355] -> w266
              tunnel: [w297 w370] -> w265
              tunnel: [w314 w369] -> w264
              tunnel: [w295 w368] -> w263
              tunnel: w261 -> [w315 w369]
              tunnel: w260 -> [_ _]
              tunnel: w259 -> [w296 w348]
              tunnel: [w296 w348] -> w258
              tunnel: [w294 w353] -> w257
              tunnel: [w292 w354] -> w256
              tunnel: w255 -> [w290 w353]
              tunnel: [w293 w349] -> w254
              tunnel: w253 -> [_ w349]
              tunnel: w252 -> [w292 w345]
              frame 0, Default {
                # "G2 gates"
                n44 = call "IMAQ Copy"("error in (no error)"=w320, "Image Dst"=w319, "Image Src"=w322) -> ("error out"=w305:errorcluster, "Image Dst Out"=w307:T2)  [unwired: 3 in]
                n45 = call "Compare Image Sizes.vi"("error in (no error)"=w305, "Image Refnum 2"=w307, "Image Refnum 1"=w309) -> ("error out"=w304:errorcluster, "Image Refnum 2 (dup)"=w306:T2, "Image Refnum 1 (dup)"=w308:T2)  [unwired: 5 in, 1 out]
                n46 = call "IMAQ Subtract"("Image Src A"=w308, "Image Dst"=w308, "Image Src B"=w306, "error in (no error)"=w304) -> ("Image Dst Out"=w297:T2, "error out"=w289:errorcluster)  [unwired: 3 in]
                n47 = call "IMAQ FillImage"("error in (no error)"=w289, "Pixel Value (U8, U16, I16, Float)"=sgl -inf, "Image"=w291) -> ("error out"=w300:errorcluster, "Image Out"=w301:T2)  [unwired: 7 in]
                n48 = call "IMAQ FillImage"("error in (no error)"=w289, "Pixel Value (U8, U16, I16, Float)"=sgl inf, "Image"=w290) -> ("error out"=w298:errorcluster, "Image Out"=w299:T2)  [unwired: 7 in]
                n49 = for {
                  tunnel: w315 -> [w339] mode=indexing
                  tunnel: w321 -> [w341] mode=indexing
                  tunnel: [w329] -> w314 mode=indexing
                  tunnel: [w325] -> w313 mode=indexing
                  tunnel: w316 -> [w342]
                  tunnel: w317 -> [w343]
                  shift-right: [w332] -> w295
                  shift-left: w301 -> [w333]
                  tunnel: w300 -> [w328]
                  shift-right: [w330] -> w294
                  shift-left: w299 -> [w331]
                  tunnel: w298 -> [w327]
                  # "seems to fix a bug"
                  n50 = call "IMAQ Copy"("error in (no error)"=w342, "Image Dst"=w343, "Image Src"=w341) -> ("error out"=w337:errorcluster, "Image Dst Out"=w338:T2)  [unwired: 3 in]
                  n51 = call "Compare Image Sizes.vi"("error in (no error)"=w337, "Image Refnum 2"=w338, "Image Refnum 1"=w339) -> ("error out"=w336:errorcluster, "Image Refnum 2 (dup)"=w334:T2, "Image Refnum 1 (dup)"=w335:T2)  [unwired: 5 in, 1 out]
                  n52 = Wait (ms)(milliseconds to wait=u32 0) -> ()  [unwired: 1 out]
                  n53 = call "IMAQ Subtract"("Image Src A"=w335, "Image Dst"=w335, "Image Src B"=w334, "error in (no error)"=w336) -> ("Image Dst Out"=w329:T2, "error out"=w323:errorcluster)  [unwired: 3 in]
                  n54 = call "Compute Max Image.vi"("error in (no error)"=w328, "New Image"=w329, "Max Image Dst"=w333) -> ("error out"=w326:errorcluster, "Max Image"=w332:T2)  [unwired: 7 in]
                  n55 = call "Compute Min Image.vi"("error in (no error)"=w327, "New Image"=w329, "Min Image Dst"=w331) -> ("error out"=w324:errorcluster, "Min Image"=w330:T2)  [unwired: 7 in]
                  n56 = Merge Errors(w326, w324, w323) -> (w325:errorcluster)
                }
                n57 = Merge Errors(w313) -> (w293:errorcluster)
              }
              frame 1 {
                # "INT gates"
                n58 = call "IMAQ Copy"("error in (no error)"=w378, "Image Dst"=w367, "Image Src"=w375) -> ("error out"=w363:errorcluster, "Image Dst Out"=w364:T2)  [unwired: 3 in]
                n59 = call "Compare Image Sizes.vi"("error in (no error)"=w363, "Image Refnum 2"=w364, "Image Refnum 1"=w365) -> ("error out"=w360:errorcluster, "Image Refnum 2 (dup)"=w361:T2, "Image Refnum 1 (dup)"=w362:T2)  [unwired: 5 in, 1 out]
                n60 = call "IMAQ Subtract"("Image Src A"=w362, "Image Dst"=w362, "Image Src B"=w361, "error in (no error)"=w360) -> ("Image Dst Out"=w352:T2, "error out"=w344:errorcluster)  [unwired: 3 in]
                n61 = call "IMAQ FillImage"("error in (no error)"=w344, "Pixel Value (U8, U16, I16, Float)"=sgl -inf, "Image"=w346) -> ("error out"=w350:errorcluster, "Image Out"=w357:T2)  [unwired: 7 in]
                n62 = call "IMAQ FillImage"("error in (no error)"=w344, "Pixel Value (U8, U16, I16, Float)"=sgl inf, "Image"=w345) -> ("error out"=w351:errorcluster, "Image Out"=w356:T2)  [unwired: 7 in]
                n63 = for {
                  tunnel: w373 -> [w395] mode=indexing
                  tunnel: w374 -> [w397] mode=indexing
                  tunnel: [w387] -> w371 mode=indexing
                  tunnel: [w381] -> w372 mode=indexing
                  tunnel: w376 -> [w398]
                  tunnel: w377 -> [w399]
                  shift-right: [w385] -> w355
                  shift-left: w357 -> [w386]
                  shift-right: [w383] -> w354
                  shift-left: w356 -> [w384]
                  tunnel: w351 -> [w380]
                  tunnel: w350 -> [w379]
                  # "seems to fix a bug"
                  n64 = call "IMAQ Copy"("error in (no error)"=w398, "Image Dst"=w399, "Image Src"=w397) -> ("error out"=w393:errorcluster, "Image Dst Out"=w394:T2)  [unwired: 3 in]
                  n65 = Wait (ms)(milliseconds to wait=u32 0) -> ()  [unwired: 1 out]
                  n66 = call "Compare Image Sizes.vi"("error in (no error)"=w393, "Image Refnum 2"=w394, "Image Refnum 1"=w395) -> ("error out"=w390:errorcluster, "Image Refnum 2 (dup)"=w391:T2, "Image Refnum 1 (dup)"=w392:T2)  [unwired: 5 in, 1 out]
                  n67 = call "IMAQ Subtract"("Image Src A"=w392, "Image Dst"=w392, "Image Src B"=w391, "error in (no error)"=w390) -> ("Image Dst Out"=w387:T2, "error out"=w382:errorcluster)  [unwired: 3 in]
                  n68 = call "Compute Max Image.vi"("error in (no error)"=w379, "New Image"=w387, "Max Image Dst"=w386) -> ("error out"=w389:errorcluster, "Max Image"=w385:T2)  [unwired: 7 in]
                  n69 = call "Compute Min Image.vi"("error in (no error)"=w380, "New Image"=w387, "Min Image Dst"=w384) -> ("error out"=w388:errorcluster, "Min Image"=w383:T2)  [unwired: 7 in]
                  n70 = Merge Errors(w389, w388, w382) -> (w381:errorcluster)
                }
                n71 = Merge Errors(w372) -> (w366:errorcluster)
              }
            }
          }
        }
      }
      n72 = in-place-cluster #2("Current Dataset Images 1.SGL Min Image"=w71, "Current Dataset Images 2.SGL Min Image"=w72, "Dual-Channel Background Dataset"=w88, "Dual-Channel Dataset"=w87, "Current Dataset Images 1.SGL Sum Image"=w97, "Current Dataset Images 1.SGL Gate Images"=w96, "Current Dataset Images 1.SGL Max Image"=w95, "Current Dataset Images 2.SGL Sum Image"=w92, "Current Dataset Images 2.SGL Gate Images"=w91, "Current Dataset Images 2.SGL Max Image"=w90) -> (w48:T5)
    }
    n73 = in-place-dvr #1(w48) -> (→"AlliGator IV DVR out":refnum<data-value>, w14:errorcluster)
  }
  n74 = Build Array(w31, w28, w26, w2) -> (w29:T2[])
  n75 = call "Tiny Clear Error.vi"("Error In"=w14) -> ("no Error Out"=w23:errorcluster)  [unwired: 8 in]
  n76 = Merge Errors(w14, w35, w34, w36) -> (w16:errorcluster)
  n77 = call "Dispose Array of Images.vi"("Array of Images"=w29, "error in (no error)"=w23) -> ()  [unwired: 7 in, 1 out]
  n78 = call <vilib>:"Clear Errors.vi"("error in (no error)"=w16, "specific error code to clear (0: all)"=-1074396120) -> ("error out"=→"error out":errorcluster)  [unwired: 4 in, 1 out]
